vi "SetPhysicalTrigger.vi"(8 "error in (no error)":errorcluster, 11 "TektronixDPO in":refnum<class "TektronixDPO.lvclass">) -> (0 "error out":errorcluster, 3 "TektronixDPO out":refnum<class "TektronixDPO.lvclass">)   [LabVIEW 2013, in "TektronixDPO.lvclass"]
doc: "Send the selected trigger settings to the physical device"
uses:
  TektronixDPO.lvclass
  TektronixDPO.lvclass/TektronixDPO.ctl
  Tektronix DPO MSO 2000 4000 Series/Public/Configure/Configure Trigger (Edge).vi
  Tektronix DPO MSO 2000 4000 Series/Tektronix DPO MSO 2000 4000 Series.lvlib
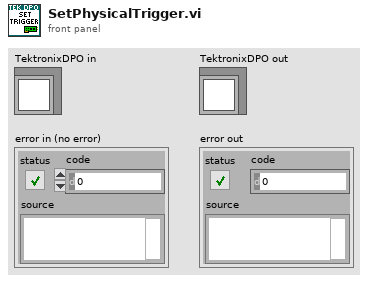
[diagram p1: front panel]
types:
  T1 = typedef "Choice73.ctl" = enum16{"Immediate", "Analog Edge"}
  T2 = typedef "Choice75.ctl" = enum16{"DC", "HF Reject", "LF Reject", "Noise Reject", "AC"}
  T3 = typedef "Choice76.ctl" = enum16{"Rising", "Falling"}
  T4 = typedef "Choice74.ctl" = enum16{"Channel 1", "Channel 2", "Channel 3", "Channel 4", "AC Line", "Aux", "Digital Channel 0", "Digital Channel 1", "Digital Channel 2", "Digital Channel 3", "Digital Channel 4", "Digital Channel 5", "Digital Channel 6", "Digital Channel 7", "Digital Channel 8", "Digital Channel 9", "Digital Channel 10", "Digital Channel 11", "Digital Channel 12", "Digital Channel 13", "Digital Channel 14", "Digital Channel 15", "RF"}
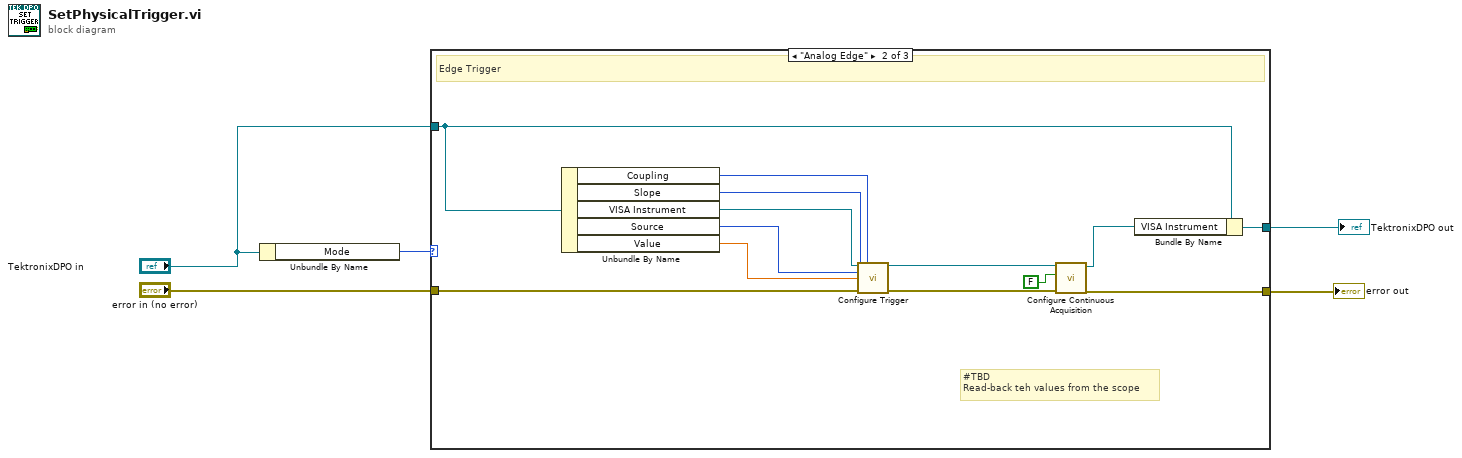
[diagram p0: block diagram]
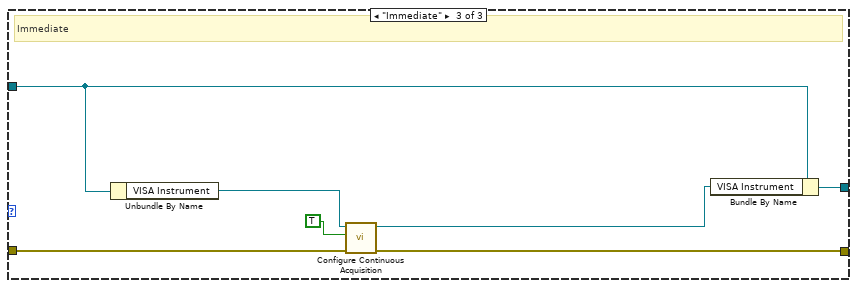
[diagram p3: hidden frame]
diagram:
  n1 = Unbundle By Name("TektronixDPO in") -> ("Mode"=w1:T1)
  n2 = case shown="\"Analog Edge\"" w1 {
    tunnel: "error in (no error)" -> [w7 w11 w26]
    tunnel: [w7 w18 w21] -> w3
    tunnel: "TektronixDPO in" -> [w6 w20 w24]
    tunnel: [w6 w19 w23] -> w5
    frame Default {
    }
    frame "Analog Edge" {
      # "#TBD\nRead-back teh values from the scope"
      # "Edge Trigger"
      n3 = Unbundle By Name(w20) -> ("Coupling"=w13:T2, "Slope"=w10:T3, "VISA Instrument"=w8:refnum<visa-resource-name>, "Source"=w9:T4, "Value"=w12:dbl)
      n4 = call-poly "Configure Trigger.vi"("VISA resource name"=w8, "Trigger Coupling (0 : DC)"=w13, "Trigger Source (0: Channel 1)"=w9, "Trigger Level (0.0 V)"=w12, "Trigger Slope (0: Rising)"=w10, "error in (no error)"=w11) -> ("VISA resource name out"=w15:refnum<visa-resource-name>, "error out"=w14:errorcluster)  [unwired: 8 in]
      n5 = call "Configure Continuous Acquisition.vi"("error in (no error)"=w14, "Enable Continuous Acquisition Mode (T: Enable)"=FALSE, "VISA resource name"=w15) -> ("error out"=w18:errorcluster, "VISA resource name out"=w16:refnum<visa-resource-name>)  [unwired: 7 in]
      n6 = Bundle By Name(cluster=w20, "VISA Instrument"=w16) -> (w19:refnum<class "TektronixDPO.lvclass">)
    }
    frame "Immediate" {
      # "Immediate"
      n7 = Unbundle By Name(w24) -> ("VISA Instrument"=w25:refnum<visa-resource-name>)
      n8 = call "Configure Continuous Acquisition.vi"("error in (no error)"=w26, "Enable Continuous Acquisition Mode (T: Enable)"=TRUE, "VISA resource name"=w25) -> ("error out"=w21:errorcluster, "VISA resource name out"=w22:refnum<visa-resource-name>)  [unwired: 7 in]
      n9 = Bundle By Name(cluster=w24, "VISA Instrument"=w22) -> (w23:refnum<class "TektronixDPO.lvclass">)
    }
  }
  "TektronixDPO out" <- w5
  "error out" <- w3
